vi "数据导入工具-main.vi"() -> ()   [LabVIEW 2016]
uses:
  <vilib>/Utility/sysdir.llb/System Directory Type.ctl
  <vilib>/addons/database/Connection.llb/DB Tools Open Connec (String).vi
  <vilib>/addons/database/NI_Database_API.lvlib
panel:
  out "selected path":path caption="所选路径"
  in  "导入日志":string
  in  "导入SQLite":bool
  in  "ACCESS数据表":bool
  in  "列表框":i32[](listbox)
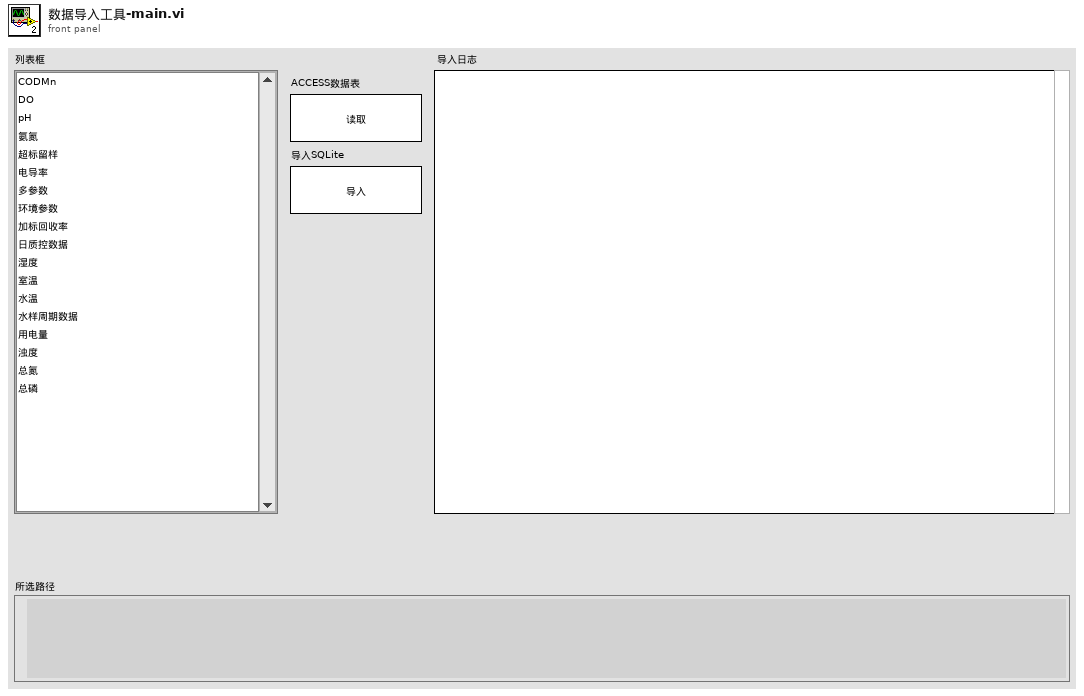
[diagram p1: front panel]
types:
  T1 = typedef "System Directory Type.ctl" = i32
  T2 = typedef "NI_Database_API.lvlib/Conn ObjectReference.ctl" = refnum<k1>
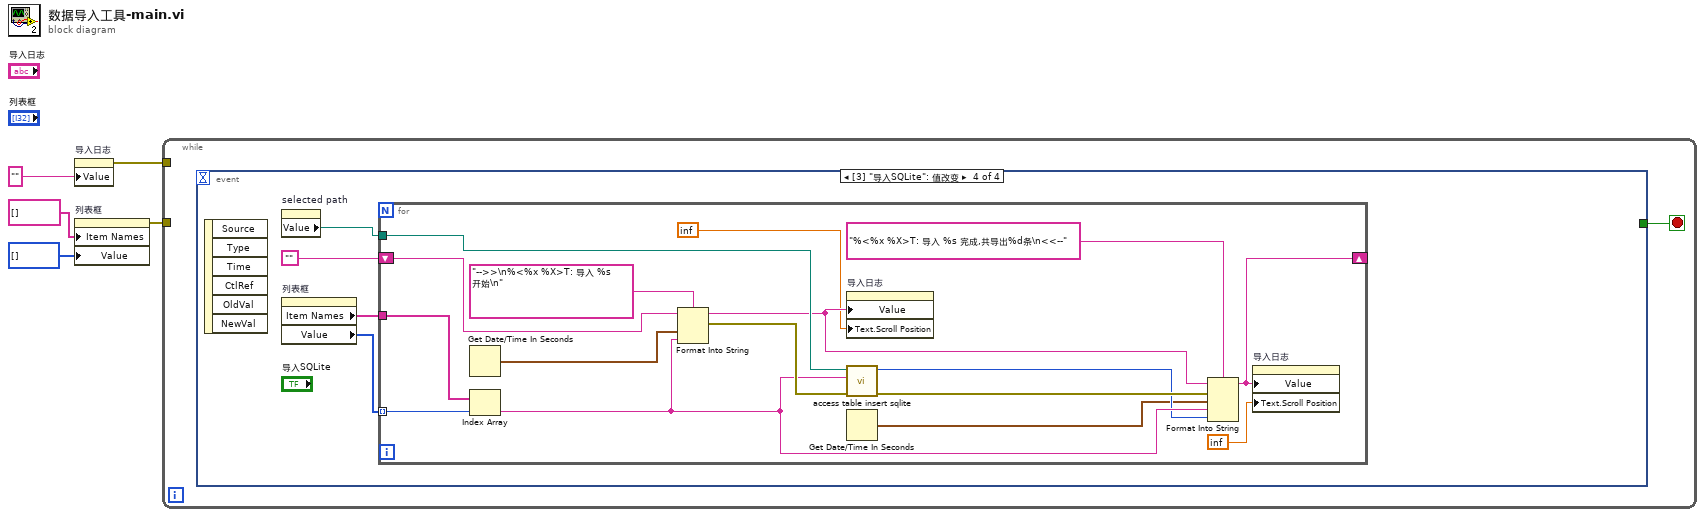
[diagram p0: block diagram]
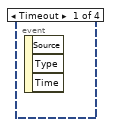
[diagram p2: hidden frame]
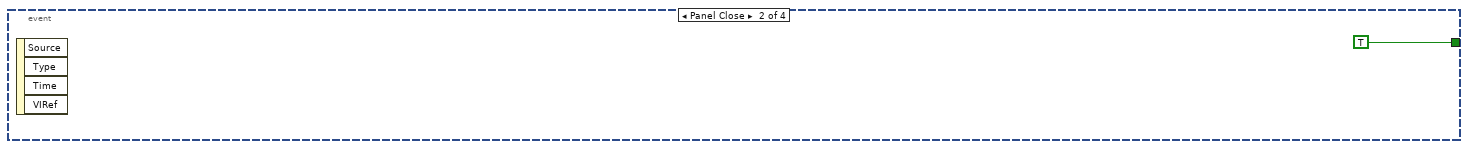
[diagram p3: hidden frame]
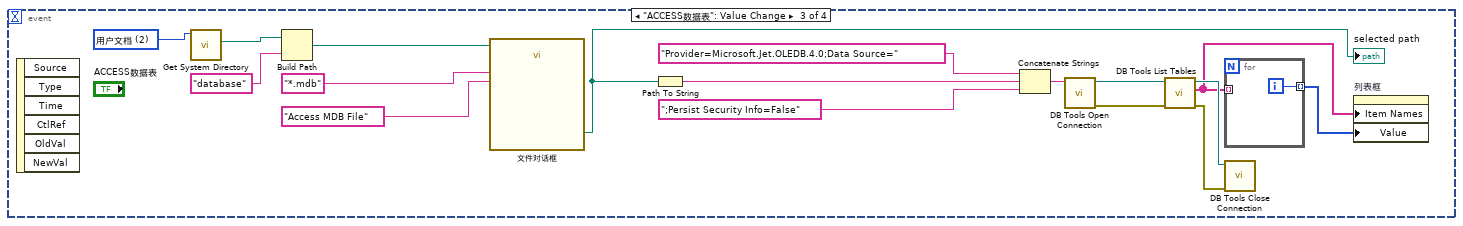
[diagram p4: hidden frame]
diagram:
  n1 = property on="导入日志" class="Str"("Value"="" ("导入日志")) -> (error out=w1:errorcluster)  [unwired: 2 in, 1 out]
  n2 = property on="列表框" class="LstBox (严格)"("Item Names"=string[] [] ("项名"), "Value"=i32[] [] ("列表框")) -> (error out=w3:errorcluster)  [unwired: 2 in, 1 out]
  n3 = while {
    tunnel: w3 -> [_]
    tunnel: w1 -> [_]
    stop <- w6 stop-if-true
    n4 = event shown="[3] \"导入SQLite\": 值改变" {
      selector: _ -> [_ _ _ _]
      dyn-events: _ -> [_ _ _ _]
      timeout: _ -> [_ _ _ _]
      tunnel: [_ TRUE _ _] -> w6
      event Timeout {
        n5 = event-data() -> ()  [unwired: 1 in, 3 out]
      }
      event Panel Close {
        n6 = event-data() -> ()  [unwired: 1 in, 4 out]
      }
      event "ACCESS数据表": Value Change {
        w24 = T1 2 items=["用户目录"=0, "用户桌面"=1, "用户文档"=2, "用户应用程序数据"=3, "用户设置"=4, "用户临时目录"=5, "公共文档"=6, "公共应用程序数据"=7, "公共设置"=8, "公共缓存"=13, "系统核心库"=9, "系统安装库"=10, "应用程序文件"=11, "启动盘根目录"=12] ("system directory type")
        n7 = event-data() -> ()  [unwired: 1 in, 6 out]
        n8 = call <vilib>:"Get System Directory.vi"("system directory type"=w24) -> ("system directory"=w23:path)  [unwired: 10 in]
        n9 = Build Path(base path=w23, name or relative path="database" ("名称或相对路径")) -> (appended path=w22:path)
        n10 = call "文件对话框"("start path"=w22, "pattern (all files)"="*.mdb", "pattern label"="Access MDB File") -> ("selected path"=w12:path)  [unwired: 9 in, 3 out]
        "selected path" <- w12
        n11 = Path To String(path=w12) -> (string=w14:string)
        n12 = Concatenate Strings("Provider=Microsoft.Jet.OLEDB.4.0;Data Source=" ("condition"), w14, ";Persist Security Info=False" ("condition")) -> (w16:string)
        n13 = call-poly <vilib>:"DB Tools Open Connection.vi"("connection information"=w16) -> ("error out"=w18:errorcluster, "connection reference"=w17:T2)  [unwired: 7 in]
        n14 = call <vilib>:"DB Tools List Tables.vi"("error in (no error)"=w18, "connection reference"=w17) -> ("error out"=w10:errorcluster, "tables"=w9:string[], "connection reference out"=w11:T2)  [unwired: 3 in]
        n15 = for {
          tunnel: w9 -> [_] mode=indexing
          tunnel: [w25] -> w8 mode=indexing
          i -> [w25]
        }
        n16 = call <vilib>:"DB Tools Close Connection.vi"("error in (no error)"=w10, "connection reference"=w11) -> ()  [unwired: 5 in, 1 out]
        n17 = property on="列表框" class="LstBox (严格)"("Item Names"=w9, "Value"=w8) -> ()  [unwired: 2 in, 2 out]
      }
      event "导入SQLite": Value Change {
        n18 = event-data() -> ()  [unwired: 1 in, 6 out]
        n19 = property on="selected path" class="Path"() -> ("Value"=w29:path)  [unwired: 2 in, 2 out]
        n20 = property on="列表框" class="LstBox (严格)"() -> ("Item Names"=w27:string[], "Value"=w28:i32[])  [unwired: 2 in, 2 out]
        n21 = for {
          tunnel: w27 -> [w45]
          tunnel: w28 -> [w44] mode=indexing
          tunnel: w29 -> [w43]
          shift-right: [w37] -> _
          shift-left: "" -> [w42]
          n22 = Get Date/Time In Seconds() -> (seconds since 1Jan1904=w34:timestamp)
          n23 = Index Array(array=w45, index=w44) -> (element=w39:string)
          n24 = Format Into String(format string="-->>\n%<%x %X>T: 导入 %s 开始\n" ("格式字符串"), initial string=w42, w34, w39) -> (resulting string=w38:string, error out=w41:errorcluster)  [unwired: 1 in]
          n25 = property on="导入日志" class="Str"("Value"=w38, "Text.Scroll Position"=inf) -> ()  [unwired: 2 in, 2 out]
          n26 = call "access table insert sqlite.vi"("error in (no error)"=w41, "table"=w39, "路径"=w43) -> ("错误输出"=w40:errorcluster, "条数"=w36:i32)  [unwired: 7 in]
          n27 = Get Date/Time In Seconds() -> (seconds since 1Jan1904=w31:timestamp)
          n28 = Format Into String(format string="%<%x %X>T: 导入 %s 完成,共导出%d条\n<<--" ("格式字符串"), initial string=w38, error in=w40, w31, w39, w36) -> (resulting string=w37:string)  [unwired: 1 out]
          n29 = property on="导入日志" class="Str"("Value"=w37, "Text.Scroll Position"=inf) -> ()  [unwired: 2 in, 2 out]
        }
      }
    }
  }
